vi "Posicion_auto.vi"() -> ()   [LabVIEW 2020]
panel:
  in  "Posicion del auto":i32=108 min=108 max=1260
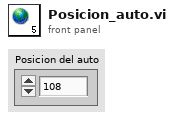
[diagram p1: front panel]
diagram:
